vi "GetInitStatus.vi"(8 "error in (no error)":errorcluster caption="错误输入（无错误）", 10 "通道选择":string="CHAN1", 11 "VISA资源名称输入":refnum<visa-resource-name>) -> (0 "error out":errorcluster caption="错误输出", 2 "读取缓冲区":string, 3 "VISA资源名称输出":refnum<visa-resource-name>)   [LabVIEW 2018]
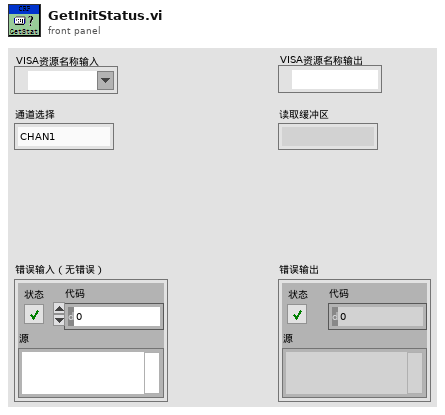
[diagram p1: front panel]
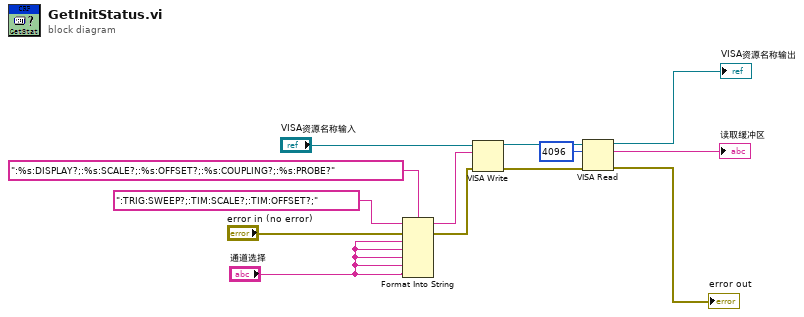
[diagram p0: block diagram]
diagram:
  n1 = Format Into String(format string=":%s:DISPLAY?;:%s:SCALE?;:%s:OFFSET?;:%s:COUPLING?;:%s:PROBE?" ("格式字符串"), initial string=":TRIG:SWEEP?;:TIM:SCALE?;:TIM:OFFSET?;", error in="error in (no error)", "通道选择", "通道选择", "通道选择", "通道选择", "通道选择") -> (resulting string=w10:string, error out=w3:errorcluster)
  n2 = VISA Write(VISA resource name="VISA资源名称输入", write buffer=w10, error in (no error)=w3) -> (VISA resource name out=w9:refnum<visa-resource-name>, error out=w8:errorcluster)  [unwired: 1 out]
  n3 = VISA Read(VISA resource name=w9, byte count=u32 4096 ("字节总数"), error in (no error)=w8) -> (VISA resource name out=→"VISA资源名称输出":refnum<visa-resource-name>, read buffer=→"读取缓冲区":string, error out=→"error out":errorcluster)  [unwired: 1 out]
